vi "InitializeEntities.vi"(8 "error in (no error)":errorcluster, 11 "client handle":T1) -> (0 "error out":errorcluster, 3 "Refnum out":T1)   [LabVIEW 2018]
uses:
  <vilib>/httpClient/ClientHandle.ctl
  <vilib>/Utility/file.llb/Read Delimited Spreadsheet (string).vi
  <vilib>/httpClient/POSTBuffer.vi
  <vilib>/httpClient/LabVIEWHTTPClient.lvlib
panel:
  out "body":string
  out "headers":string
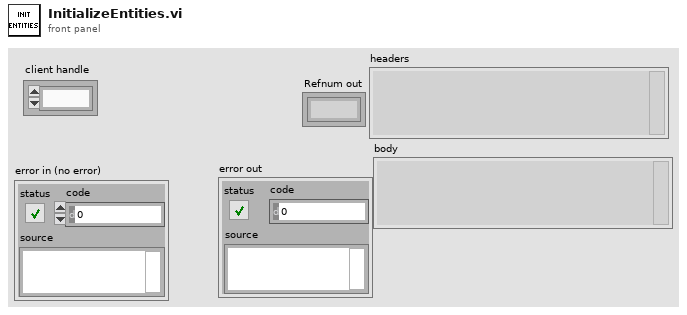
[diagram p1: front panel]
types:
  T1 = typedef "LabVIEWHTTPClient.lvlib/ClientHandle.ctl" = refnum<k1>
  T2 = cluster{"ID":string, "Date":string, "StreetAddress":string, "longitude":string, "latitude":string, "Device":string, "Index":string}
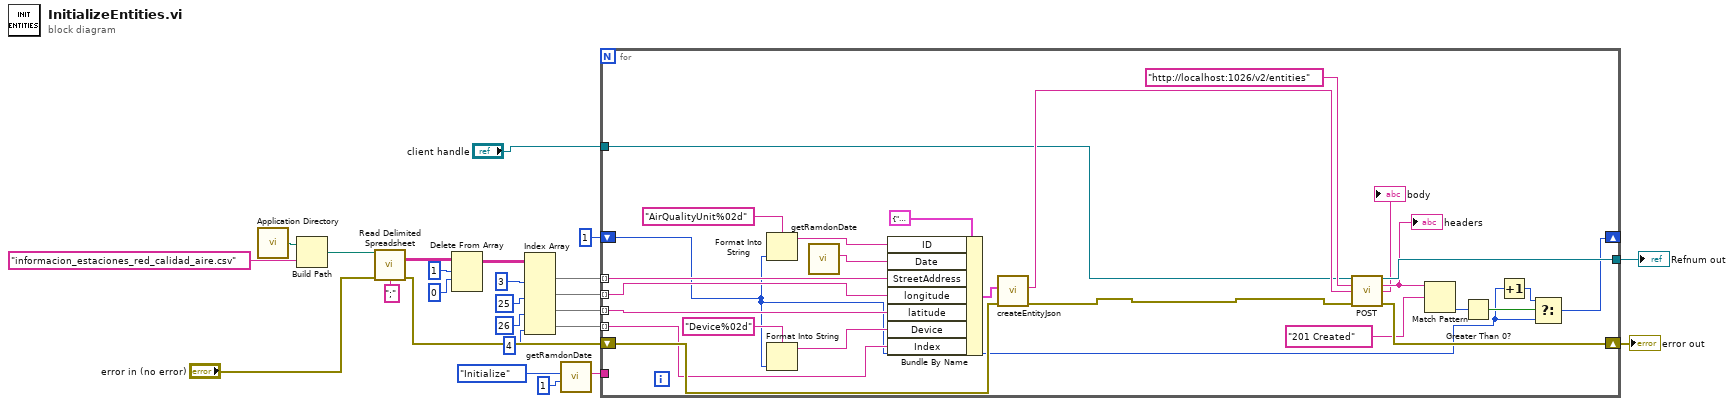
[diagram p0: block diagram]
diagram:
  n1 = call <vilib>:"Application Directory.vi"() -> ("Application Directory"=w8:path)
  n2 = Build Path(base path=w8, name or relative path="informacion_estaciones_red_calidad_aire.csv") -> (appended path=w10:path)
  n3 = call-poly <vilib>:"Read Delimited Spreadsheet.vi"("file path (dialog if empty)"=w10, "error in (no error)"="error in (no error)", "delimiter (\\t)"=";" ("delimiter (\\t)")) -> ("all rows"=w20:string[][], "error out"=w6:errorcluster)  [unwired: 7 in, 4 out]
  n4 = Delete From Array(array=w20, length=1, index (row)=0) -> (array with subset deleted=w23:string[][])  [unwired: 1 in, 1 out]
  n5 = Index Array(array=w23, index (col) #1=3 ("disabled index (col)"), index (col) #2=25 ("index (col)"), index (col) #3=26 ("index (col)"), index (col) #4=4 ("index (col)")) -> (element #1=w17:string[], element #2=w18:string[], element #3=w19:string[], element #4=w2:string[])  [unwired: 4 in]
  n6 = call "getRamdonDate.vi"("Start Day"=1, "Action (GetDate)"=enum16{"Initialize", "GetDate"}."Initialize") -> ("Ramdon date"=w24:string)  [unwired: 9 in]
  n7 = for {
    tunnel: w17 -> [w50] mode=indexing
    tunnel: w18 -> [w46] mode=indexing
    tunnel: w19 -> [w45] mode=indexing
    tunnel: w24 -> [_]
    tunnel: [w41] -> w25
    shift-right: [w39] -> w5
    shift-left: w6 -> [w40]
    shift-right: [w35] -> _
    shift-left: 1 ("offset past match") -> [w30]
    tunnel: w2 -> [w31] mode=indexing
    tunnel: "client handle" -> [w26]
    n8 = Format Into String(format string="AirQualityUnit%02d", w30) -> (resulting string=w47:string)  [unwired: 2 in, 1 out]
    n9 = Format Into String(format string="Device%02d", w30) -> (resulting string=w49:string)  [unwired: 2 in, 1 out]
    n10 = call "getRamdonDate.vi"() -> ("Ramdon date"=w42:string)  [unwired: 11 in]
    n11 = Bundle By Name(cluster=T2 {"ID"="AirQualityUnit24", "Date"="2021-01-1T16:10:27-02:00", "StreetAddress"="Plaza Tres Olivos ", "longitude"="-3.6897308", "latitude"="40.5005477", "Device"="Device24", "Index"="45"} ("Data"), "ID"=w47, "Date"=w42, "StreetAddress"=w50, "longitude"=w46, "latitude"=w45, "Device"=w49, "Index"=w31) -> (w32:T2)
    n12 = call "createEntityJson.vi"("error in (no error)"=w40, "Data"=w32) -> ("error out"=w27:errorcluster, "AirQualityObservedEntity"=w43:string)  [unwired: 8 in]
    n13 = call-poly <vilib>:"POST.vi"("client handle"=w26, "url"="http://localhost:1026/v2/entities", "buffer"=w43, "error in (no error)"=w27) -> ("client handle out"=w41:T1, "headers"=w29:string, "body"=→"body":string, "error out"=w39:errorcluster)  [unwired: 8 in]
    "headers" <- w29
    n14 = Match Pattern(string=w29, regular expression="201 Created") -> (offset past match=w37:i32)  [unwired: 1 in, 3 out]
    n15 = Greater Than 0?(x=w37) -> (x > 0?=w36:bool)
    n16 = Increment(x=w30) -> (x+1=w34:i32)
    n17 = Select(t=w34, s=w36, f=w30) -> (s? t:f=w35:i32)
  }
  "Refnum out" <- w25
  "error out" <- w5
